vi "题目7.vi"() -> ()   [LabVIEW 2017]
panel:
  out "所用时间（ms）":u32
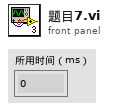
[diagram p1: front panel]
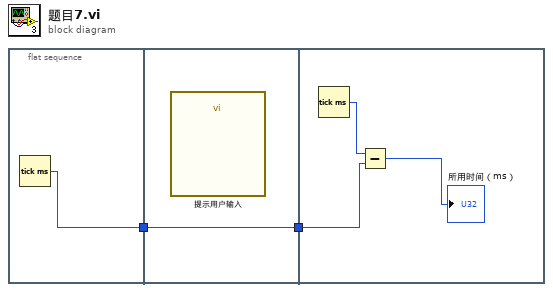
[diagram p0: block diagram]
diagram:
  n1 = flat-sequence {
    tunnel: [w3] -> w2
    tunnel: w2 -> [w4]
    tunnel: [w4] -> w1
    tunnel: w1 -> [w7]
    frame #0 {
      n2 = Tick Count (ms)() -> (millisecond timer value=w3:u32)
    }
    frame #1 {
      n3 = call "提示用户输入"() -> ()  [unwired: 16 in, 4 out]
    }
    frame #2 {
      n4 = Tick Count (ms)() -> (millisecond timer value=w6:u32)
      n5 = Subtract(x=w6, y=w7) -> (x-y=→"所用时间（ms）":u32)
    }
  }
